vi "sub_list_all_channels_for_device.vi"(8 "error in (no error)":errorcluster, 11 "daq.io type in":T1={"daq.io ref"=refnum, "daq.io API Base"="http://dashboard.daq.io/api/v1", "Device Key"="", "Account ID"="", "online"=TRUE, "SSL"=FALSE}) -> (0 "error out":errorcluster, 2 "List of Channel Keys":string[](array[string]), 3 "daq.io type out":T1={"daq.io ref"=refnum, "daq.io API Base"="http://dashboard.daq.io/api/v1", "Device Key"="", "Account ID"="", "online"=TRUE, "SSL"=FALSE})   [LabVIEW 2013, in "daqio minimal.lvlib"]
doc: "This VI list all Channels for a specified Device"
uses:
  daqio minimal.lvlib
  _typedefs/daqio-Type.ctl
  <vilib>/httpClient/ClientHandle.ctl
  _typedefs/daqio-Device.ctl
  _typedefs/daqio-Channels.ctl
  _typedefs/daqio-Device-Dashboards.ctl
  <vilib>/Easy HTTP Client/Easy HTTP.lvlib
  <vilib>/httpClient/LabVIEWHTTPClient.lvlib
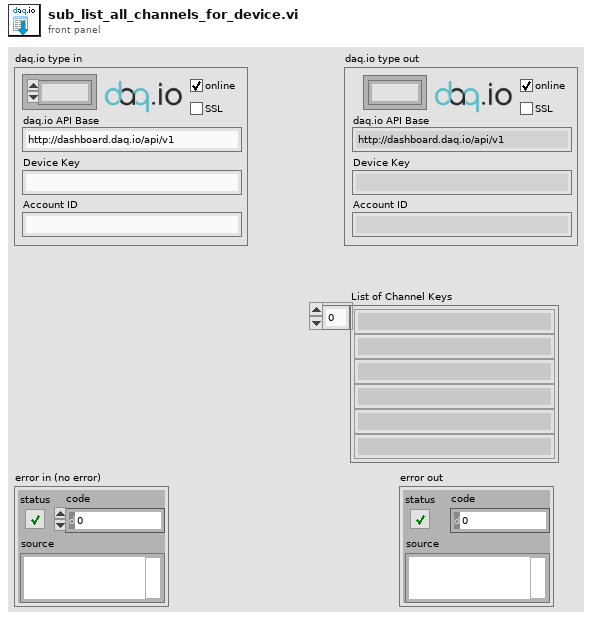
[diagram p1: front panel]
types:
  T1 = typedef "daqio minimal.lvlib/daqio-Type.ctl" = cluster{"daq.io ref":T2, "daq.io API Base":string, "Device Key":string, "Account ID":string, "online":bool, "SSL":bool}
  T2 = typedef "LabVIEWHTTPClient.lvlib/ClientHandle.ctl" = refnum<k1>
  T3 = typedef "daqio minimal.lvlib/daqio-Device.ctl" = cluster{"id":string, "label":string, "key":string, "channels":T4[], "tags":cluster{"key":string, "value":string}[], "events":cluster{"id":string, "key":string, "label":string}[], "files":string[], "permissions":cluster{"write":string[], "read":string[]}, "dashboards":T5[]}
  T4 = typedef "daqio minimal.lvlib/daqio-Channels.ctl" = cluster{"key":string, "label":string, "data_type":string, "id":string}
  T5 = typedef "daqio-Device-Dashboards.ctl" = cluster{"active":bool, "definition":string, "_id":string, "label":string}
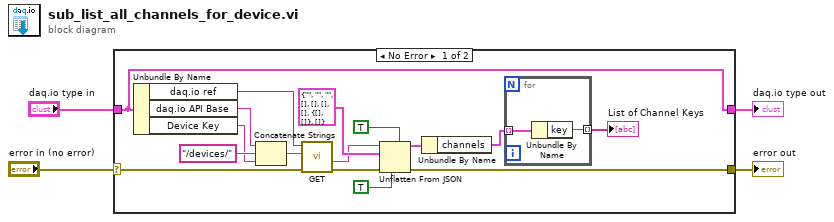
[diagram p0: block diagram]
diagram:
  n1 = case shown="No Error" "error in (no error)" {
    selector: "error in (no error)" -> [w14 w23]
    tunnel: [w7 w23] -> w3
    tunnel: "daq.io type in" -> [w6 w24]
    tunnel: [w6 w24] -> w1
    frame No Error {
      n2 = Unbundle By Name(w6) -> ("daq.io ref"=w19:T2, "daq.io API Base"=w18:string, "Device Key"=w16:string)
      n3 = Concatenate Strings(w18, "/devices/" ("string"), w16) -> (w15:string)
      n4 = call <vilib>:"GET.vi"("error in (no error)"=w14, "url"=w15, "client handle"=w19) -> ("error out"=w20:errorcluster, "body"=w12:string)  [unwired: 4 in, 3 out]
      n5 = Unflatten From JSON(enable LabVIEW extensions? (T)=TRUE, JSON string=w12, type and defaults=T3 {"id"="", "label"="", "key"="", "channels"=[], "tags"=[], "events"=[], "files"=[], "permissions"={"write"=[], "read"=[]}, "dashboards"=[]} ("Device"), default null elements? (F)=TRUE, error in (no error)=w20) -> (value=w10:T3, error out=w7:errorcluster)  [unwired: 2 in]
      n6 = Unbundle By Name(w10) -> ("channels"=w9:T4[])
      n7 = for {
        tunnel: w9 -> [w22] mode=indexing
        tunnel: [w21] -> w8 mode=indexing
        n8 = Unbundle By Name(w22) -> ("key"=w21:string)
      }
      "List of Channel Keys" <- w8
    }
    frame Error {
    }
  }
  "error out" <- w3
  "daq.io type out" <- w1
